vi "rotateImage.vi"(0 "Input":bool[][](array[boolean])=[[FALSE, FALSE, TRUE, FALSE], [FALSE, TRUE, TRUE, FALSE], [FALSE, FALSE, TRUE, FALSE], [FALSE, FALSE, TRUE, FALSE], [TRUE, TRUE, TRUE, TRUE]]) -> (1 "rotate 90":bool[][](array[boolean]), 2 "rotate 270":bool[][](array[boolean]))   [LabVIEW 2012]
panel:
  out "transpose":bool[][](array[boolean])
  out "rotate 180":bool[][](array[boolean])
  out "Diagonal flip":bool[][](array[boolean])
  out "Horizontal  flip":bool[][](array[boolean])
  out "Vertical flip":bool[][](array[boolean])
  # "This VI shows how to apply all simple symmetry operations to a 2D array.\n\nChristian Altenbach, altenbach@gmail.com"
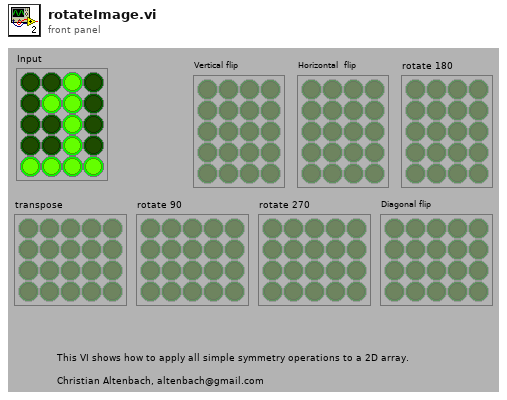
[diagram p1: front panel]
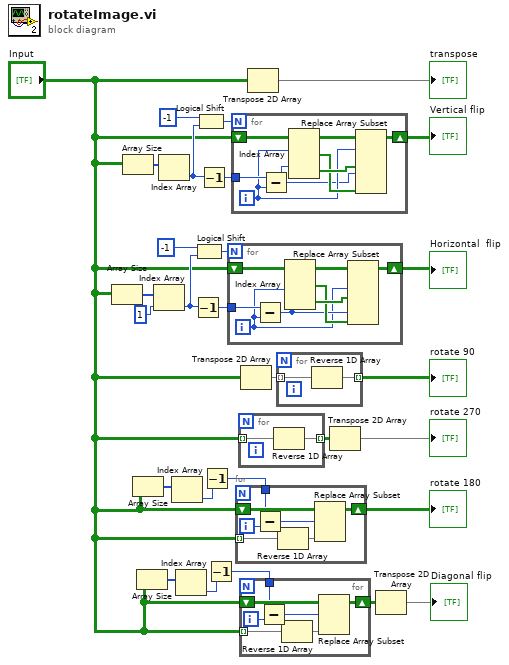
[diagram p0: block diagram]
diagram:
  n1 = Array Size(array="Input") -> (size(s)=w14:i32[])
  n2 = Array Size(array="Input") -> (size(s)=w23:i32[])
  n3 = Array Size(array="Input") -> (size(s)=w9:i32[])
  n4 = Array Size(array="Input") -> (size(s)=w4:i32[])
  n5 = Index Array(array=w14, index=1) -> (element=w16:i32)
  n6 = Index Array(array=w23) -> (element=w21:i32)  [unwired: 1 in]
  n7 = Index Array(array=w9) -> (element=w7:i32)  [unwired: 1 in]
  n8 = Index Array(array=w4) -> (element=w6:i32)  [unwired: 1 in]
  n9 = Decrement(x=w16) -> (x-1=w18:i32)
  n10 = Logical Shift(y=i8 -1, x=w16) -> (x << y=w15:i32)
  n11 = Logical Shift(y=i8 -1, x=w21) -> (x << y=w22:i32)
  n12 = Decrement(x=w21) -> (x-1=w19:i32)
  n13 = Decrement(x=w7) -> (x-1=w8:i32)
  n14 = Decrement(x=w6) -> (x-1=w5:i32)
  n15 = for {
    N: w15 -> [_]
    shift-right: [w35] -> w13
    shift-left: "Input" -> [w34]
    tunnel: w18 -> [w31]
    i -> [w29]
    n16 = Subtract(x=w31, y=w29) -> (x-y=w30:i32)
    n17 = Index Array(array=w34, index (col) #1=w29, index (col) #2=w30) -> (element #1=w32:bool[], element #2=w33:bool[])  [unwired: 2 in]
    n18 = Replace Array Subset(array=w34, new element #1=w33, index (col) #1=w29, new element #2=w32, index (col) #2=w30) -> (w35:bool[][])  [unwired: 2 in]
  }
  "Horizontal  flip" <- w13
  n19 = for {
    N: w22 -> [_]
    shift-right: [w42] -> w28
    shift-left: "Input" -> [w41]
    tunnel: w19 -> [w38]
    i -> [w37]
    n20 = Subtract(x=w38, y=w37) -> (x-y=w36:i32)
    n21 = Index Array(array=w41, index (row) #1=w37, index (row) #2=w36) -> (element #1=w39:bool[], element #2=w40:bool[])  [unwired: 2 in]
    n22 = Replace Array Subset(array=w41, new element #1=w40, index (row) #1=w37, new element #2=w39, index (row) #2=w36) -> (w42:bool[][])  [unwired: 2 in]
  }
  "Vertical flip" <- w28
  n23 = for {
    shift-right: [w49] -> w11
    shift-left: "Input" -> [w48]
    tunnel: w8 -> [w46]
    tunnel: "Input" -> [w43] mode=indexing
    i -> [w47]
    n24 = Subtract(x=w46, y=w47) -> (x-y=w45:i32)
    n25 = Reverse 1D Array(array=w43) -> (reversed array=w44:bool[])
    n26 = Replace Array Subset(array=w48, new element=w44, index (row)=w45) -> (w49:bool[][])  [unwired: 1 in]
  }
  "rotate 180" <- w11
  n27 = for {
    tunnel: "Input" -> [w51] mode=indexing
    tunnel: [w50] -> w26 mode=indexing
    n28 = Reverse 1D Array(array=w51) -> (reversed array=w50:bool[])
  }
  n29 = for {
    shift-right: [w58] -> w2
    shift-left: "Input" -> [w57]
    tunnel: w5 -> [w55]
    tunnel: "Input" -> [w52] mode=indexing
    i -> [w56]
    n30 = Subtract(x=w55, y=w56) -> (x-y=w54:i32)
    n31 = Reverse 1D Array(array=w52) -> (reversed array=w53:bool[])
    n32 = Replace Array Subset(array=w57, new element=w53, index (row)=w54) -> (w58:bool[][])  [unwired: 1 in]
  }
  n33 = Transpose 2D Array(2D array="Input") -> (transposed array=w12:bool[][])
  n34 = Transpose 2D Array(2D array="Input") -> (transposed array=→"transpose":bool[][])
  n35 = for {
    tunnel: w12 -> [w60] mode=indexing
    tunnel: [w59] -> w27 mode=indexing
    n36 = Reverse 1D Array(array=w60) -> (reversed array=w59:bool[])
  }
  "rotate 90" <- w27
  n37 = Transpose 2D Array(2D array=w26) -> (transposed array=→"rotate 270":bool[][])
  n38 = Transpose 2D Array(2D array=w2) -> (transposed array=→"Diagonal flip":bool[][])
